vi "Full Sequence Reading.vi"(8 "VISA resource name":refnum<visa-resource-name>="COM5", 9 "Delay Sample":dbl=0.001 format="%e", 10 "Save Button":bool, 11 "file path (use dialog)":path) -> (2 "VISA resource name 2":refnum<visa-resource-name>, 4 "Imag FFT":cluster{"magnitude":dbl[], dbl[]}(graph), 5 "Imag Time":cluster{"magnitude":dbl[], dbl[]}(graph), 6 "Real FFT":cluster{"magnitude":dbl[], dbl[]}(graph), 7 "Real Time":cluster{"magnitude":dbl[], dbl[]}(graph))   [LabVIEW 2011]
uses:
  <vilib>/Utility/file.llb/Write To Spreadsheet File (I64).vi
panel:
  out "error out":errorcluster
  out "Inner While":i32
  out "Outter While":i32
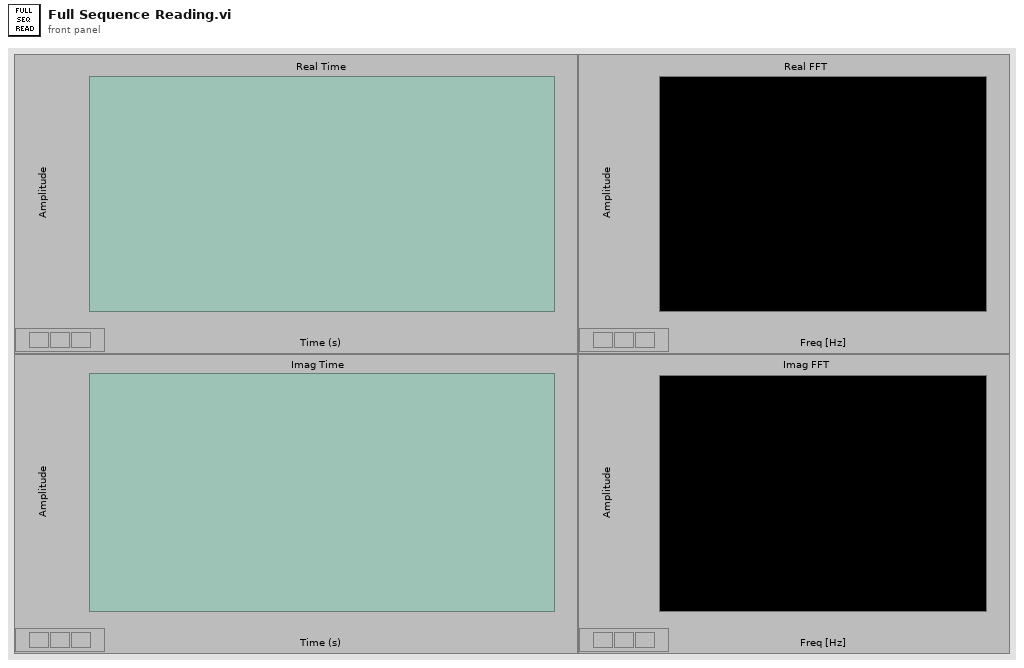
[diagram p1: front panel]
types:
  T1 = enum16{"open", "replace", "create", "open or create", "replace or create", "replace or create with confirmation"}
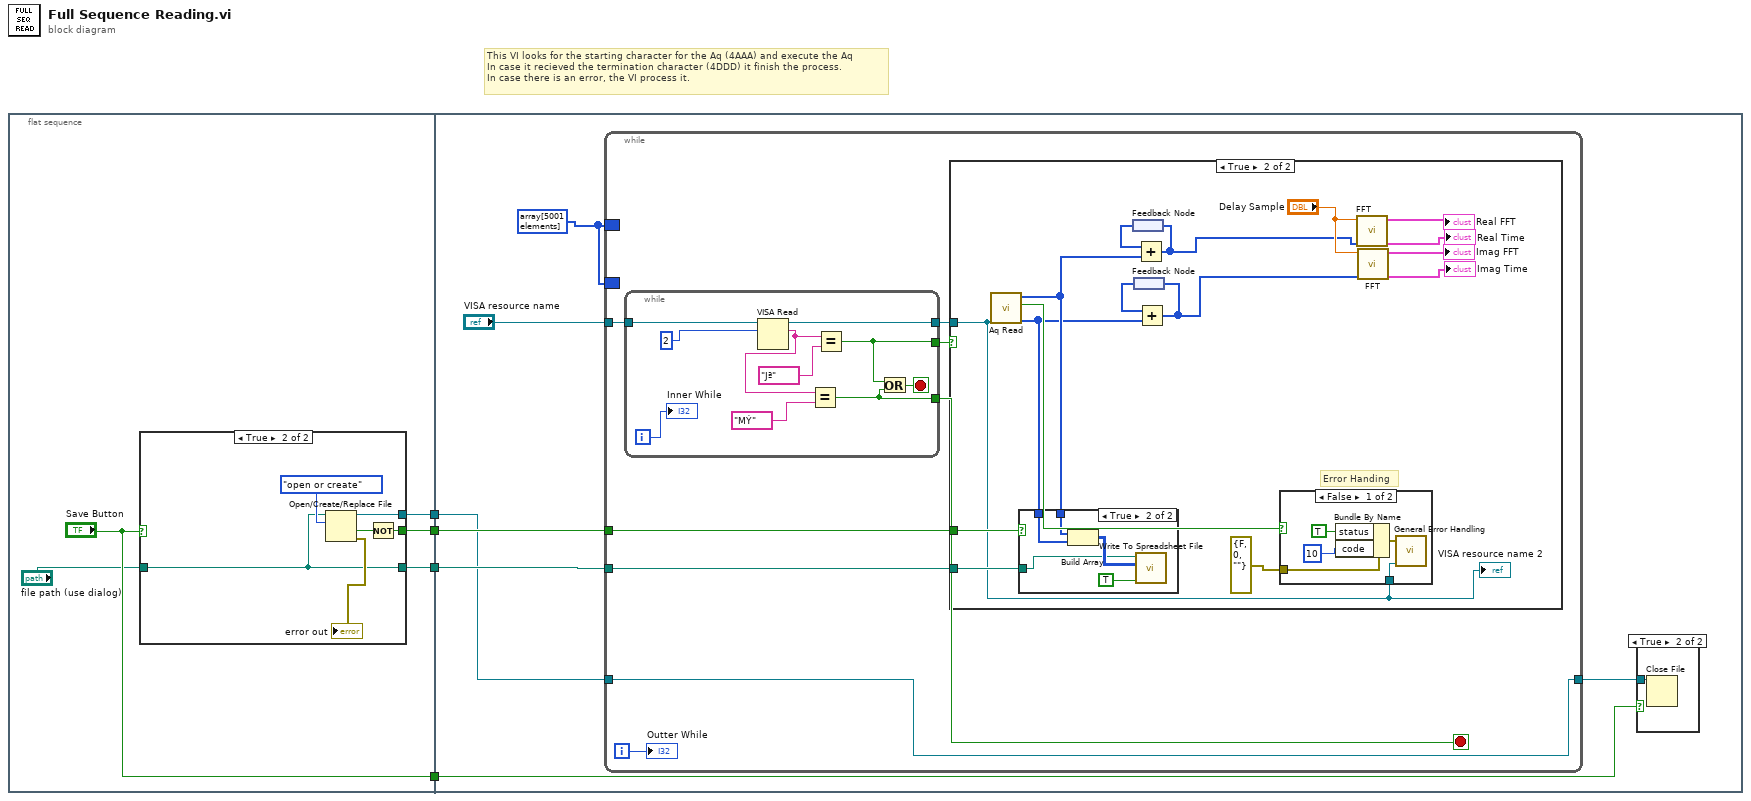
[diagram p0: block diagram]
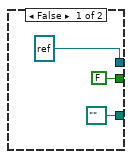
[diagram p2: hidden frame]
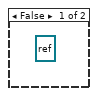
[diagram p4: hidden frame]
diagram:
  # "This VI looks for the starting character for the Aq (4AAA) and execute the Aq\nIn case it recieved the termination character (4DDD) it finish the process.\nIn case there is an error, the VI process it."
  n1 = flat-sequence {
    tunnel: [w9] -> w4
    tunnel: [w8] -> w3
    tunnel: [w7] -> w2
    tunnel: ["Save Button"] -> w1
    tunnel: w4 -> [w24]
    tunnel: w3 -> [w23]
    tunnel: w2 -> [w22]
    tunnel: w1 -> [w20]
    frame #0 {
      n2 = case shown="True" "Save Button" {
        tunnel: [FALSE w15] -> w9
        tunnel: [path "" ("appended path") w13] -> w8
        tunnel: [refnum<file> refnum ("refnum out") w14] -> w7
        tunnel: "file path (use dialog)" -> [_ w13]
        frame False {
        }
        frame True {
          n3 = Open/Create/Replace File(file path (use dialog)=w13, operation (0:open)=T1."open or create") -> (refnum out=w14:refnum<file>, cancelled=w17:bool, error out=→"error out":errorcluster)  [unwired: 4 in]
          n4 = Not(x=w17) -> (.not. x?=w15:bool)
        }
      }
    }
    frame #1 {
      w19 = i32[] array[5001 elements]
      n5 = while {
        tunnel: "VISA resource name" -> [w34]
        tunnel: w23 -> [w29]
        tunnel: w24 -> [w28]
        tunnel: w22 -> [w27]
        tunnel: [w27] -> w21
        border: w19 -> [_]
        border: w19 -> [_]
        i -> [w30]
        stop <- w32 stop-if-true
        n6 = while {
          tunnel: w34 -> [w70]
          tunnel: [w67] -> w33
          tunnel: [w63] -> w32
          tunnel: [w62] -> w31
          i -> [w61]
          stop <- w64 stop-if-true
          n7 = VISA Read(VISA resource name=w70, byte count=u32 2) -> (VISA resource name out=w67:refnum<visa-resource-name>, read buffer=w66:string)  [unwired: 1 in, 2 out]
          n8 = Equal?(x=w66, y="MÝ") -> (x = y?=w63:bool)
          n9 = Equal?(x=w66, y="Jª") -> (x = y?=w62:bool)
          n10 = Or(x=w62, y=w63) -> (x .or. y?=w64:bool)
          "Inner While" <- w61
        }
        n11 = case shown="True" w31 {
          tunnel: w33 -> [_ w45]
          tunnel: w29 -> [_ w47]
          tunnel: w28 -> [_ w48]
          frame False {
            (unwired) refnum<file> refnum ("refnum out")
          }
          frame True {
            # "Error Handing"
            n12 = call "Aq Read.vi"("VISA resource name"=w45) -> ("Imag Data"=w41:i32[], "Coincidence Of Character"=w49:bool, "Real Data"=w44:i32[])  [unwired: 7 in, 1 out]
            n13 = case shown="True" w48 {
              tunnel: w44 -> [_ w53]
              tunnel: w41 -> [_ w52]
              tunnel: w47 -> [_ w51]
              frame False {
              }
              frame True {
                n14 = Build Array(w53, w52) -> (w54:i32[][])
                n15 = call-poly <vilib>:"Write To Spreadsheet File.vi"("append to file? (new file:F)"=TRUE, "2D data"=w54, "file path (dialog if empty)"=w51) -> ()  [unwired: 5 in, 1 out]
              }
            }
            n16 = feedback #1() -> (w43:i32[])
            n17 = feedback #2() -> (w42:i32[])
            n18 = Add(x=w43, y=w44) -> (x+y=w40:i32[])
            n19 = feedback-in #1(w40) -> ()
            n20 = Add(x=w42, y=w41) -> (x+y=w39:i32[])
            n21 = feedback-in #2(w39) -> ()
            n22 = case shown="False" w49 {
              tunnel: errorcluster {"status"=FALSE, "code"=0, "source"=""} ("error out") -> [w58 _]
              tunnel: w45 -> [w56 _]
              frame False {
                n23 = Bundle By Name(cluster=w58, "status"=TRUE, "code"=10) -> (w57:errorcluster)
                n24 = call "General Error Handling.vi"("VISA resource name"=w56, "error IO"=w57) -> ()  [unwired: 10 in]
              }
              frame True {
              }
            }
            n25 = call "FFT.vi"("Input Array"=w40, "Delay Sample"="Delay Sample") -> ("Time Graph"=→"Real Time":cluster{"magnitude":dbl[], dbl[]}, "FFT Graph"=→"Real FFT":cluster{"magnitude":dbl[], dbl[]})  [unwired: 8 in]
            n26 = call "FFT.vi"("Input Array"=w39, "Delay Sample"="Delay Sample") -> ("Time Graph"=→"Imag Time":cluster{"magnitude":dbl[], dbl[]}, "FFT Graph"=→"Imag FFT":cluster{"magnitude":dbl[], dbl[]})  [unwired: 8 in]
            "VISA resource name 2" <- w45
          }
        }
        "Outter While" <- w30
      }
      n27 = case shown="True" w20 {
        tunnel: w21 -> [_ w26]
        frame False {
        }
        frame True {
          n28 = Close File(refnum=w26) -> ()  [unwired: 1 in, 2 out]
        }
      }
    }
  }
